vi "mat_2_bmp.vi"(10 "Path":path, 11 "Path 7":path) -> ()   [LabVIEW 2015]
uses:
  globala.vi
panel:
  out "x*y":i32
  out "Numeric 2":i32
  out "Numeric":i32
  out "output 2":i32
  out "output 1":i32
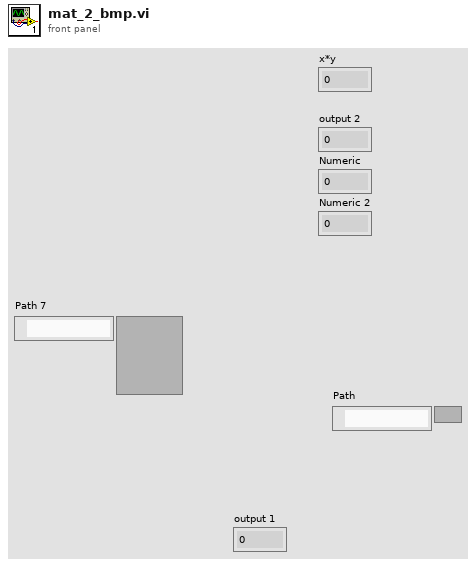
[diagram p1: front panel]
types:
  T1 = enum16{"open", "replace", "create", "open or create", "replace or create", "replace or create with confirmation"}
  T2 = typedef "imagedata.ctl" = cluster{"image type":i32, "image depth":i32, "image":u8[], "mask":u8[], "colors":u32[], "Rectangle":cluster{"left":i16, "top":i16, "right":i16, "bottom":i16}}
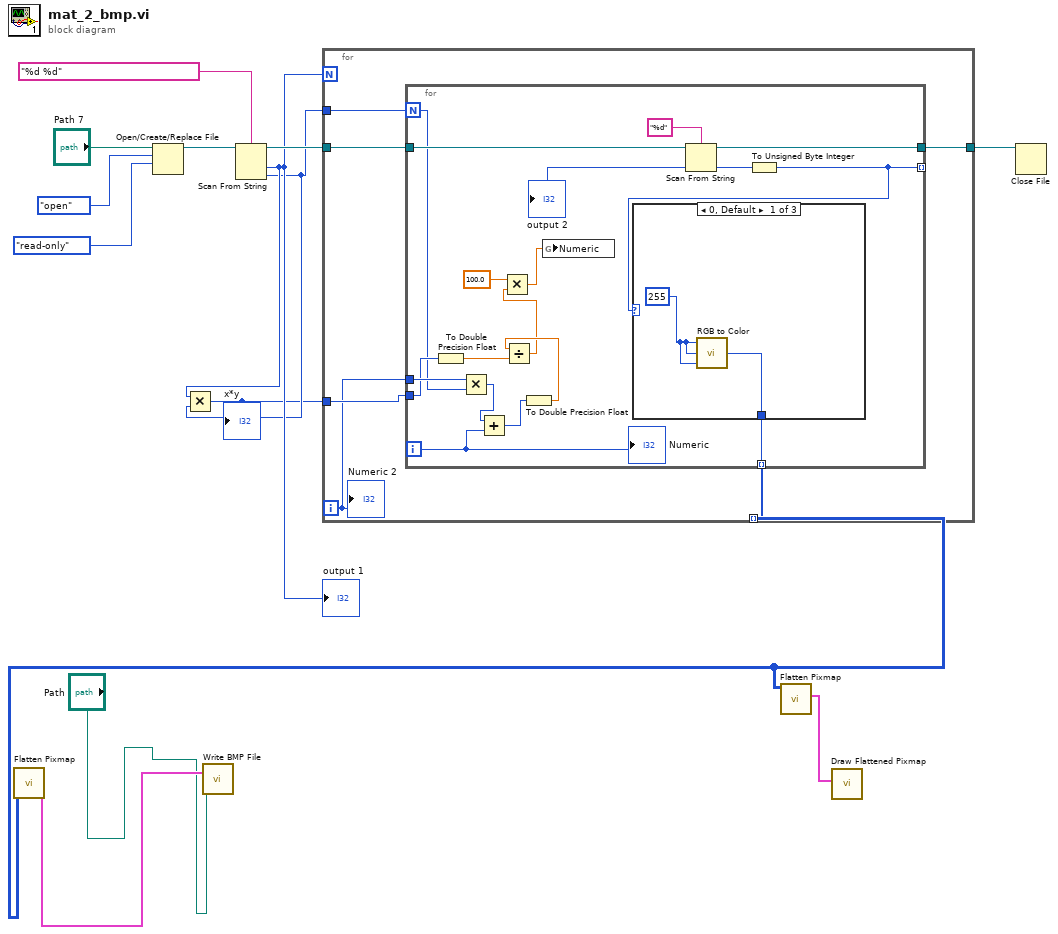
[diagram p0: block diagram]
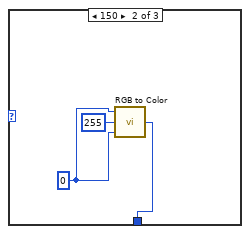
[diagram p2: hidden frame]
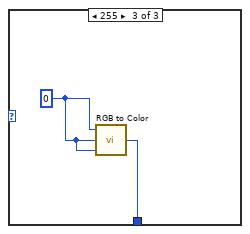
[diagram p3: hidden frame]
diagram:
  n1 = Open/Create/Replace File(file path (use dialog)="Path 7", operation (0:open)=T1."open", access (0:read/write)=enum16{"read/write", "read-only", "write-only"}."read-only") -> (refnum out=w11:refnum<file>)  [unwired: 3 in, 2 out]
  n2 = Scan From String("%d %d" ("format string"), w11) -> (w9:refnum<file>, output 1=w3:i32, output 2=w2:i32)  [unwired: 3 in, 1 out]
  "output 1" <- w3
  n3 = Multiply(x=w3, y=w2) -> (x*y=w1:i32)
  "x*y" <- w1
  n4 = for {
    N: w3 -> [_]
    tunnel: w2 -> [w20]
    tunnel: w9 -> [w19]
    tunnel: [w18] -> w8
    tunnel: [w17] -> w5 mode=indexing
    tunnel: w1 -> [w16]
    i -> [w15]
    n5 = for {
      N: w20 -> [w25]
      tunnel: w19 -> [w37]
      tunnel: [w32] -> _ mode=indexing
      tunnel: [w35] -> w18
      tunnel: [w33] -> w17 mode=indexing
      tunnel: w16 -> [w30]
      tunnel: w15 -> [w31]
      i -> [w23]
      n6 = To Double Precision Float(number=w30) -> (double precision float=w29:dbl)
      n7 = Multiply(x=w31, y=w25) -> (x*y=w24:i32)
      n8 = Add(x=w24, y=w23) -> (x+y=w22:i32)
      n9 = To Double Precision Float(number=w22) -> (double precision float=w28:dbl)
      n10 = Divide(x=w28, y=w29) -> (x/y=w27:dbl)
      n11 = Multiply(x=100.0, y=w27) -> (x*y=w21:dbl)
      n12 = global write "globala.vi" "Numeric"(w21) -> ()
      n13 = Scan From String("%d" ("format string"), w37) -> (w35:refnum<file>, output 1=w34:i32)  [unwired: 2 in, 1 out]
      "output 2" <- w34
      n14 = To Unsigned Byte Integer(number=w34) -> (unsigned 8bit integer=w32:u8)
      n15 = case shown="0, Default" w32 {
        tunnel: [w38 w40 w43] -> w33
        frame 0, Default {
          w39 = u8 255
          n16 = call <vilib>:"RGB to Color.vi"("B"=w39, "G"=w39, "R"=w39) -> ("Color"=w38:u32)
        }
        frame 150 {
          w41 = 0
          n17 = call <vilib>:"RGB to Color.vi"("B"=w41, "G"=u8 255, "R"=w41) -> ("Color"=w40:u32)
        }
        frame 255 {
          w44 = 0
          n18 = call <vilib>:"RGB to Color.vi"("B"=w44, "G"=w44, "R"=w44) -> ("Color"=w43:u32)
        }
      }
      "Numeric" <- w23
    }
    "Numeric 2" <- w15
  }
  n19 = call <vilib>:"Flatten Pixmap.vi"("24-bit pixmap"=w5) -> ("image data"=w7:T2)  [unwired: 10 in]
  n20 = call <vilib>:"Write BMP File.vi"("image data"=w7, "path to BMP file"="Path") -> ()  [unwired: 8 in, 2 out]
  n21 = call <vilib>:"Flatten Pixmap.vi"("24-bit pixmap"=w5) -> ("image data"=w4:T2)  [unwired: 10 in]
  n22 = call <vilib>:"Draw Flattened Pixmap.vi"("image data"=w4) -> ()  [unwired: 8 in, 1 out]
  n23 = Close File(refnum=w8) -> ()  [unwired: 1 in, 2 out]
